vi "MSScript_Calc_GetCmdType.vi"(2 "element":string) -> (1 "Param Items":i32, 4 "SetArray?":bool, 5 "Type":T1)   [LabVIEW 2018, in "MSScript.lvclass"]
uses:
  MSScript.lvclass
  CalcCmdType.ctl
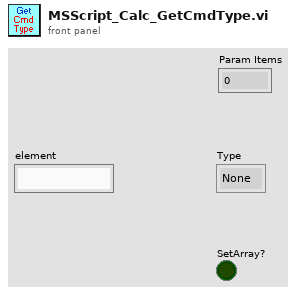
[diagram p1: front panel]
types:
  T1 = typedef "CalcCmdType.ctl" = enum16{"None", "Add", "Sub", "Multiply", "Div", "Pow", "Mod", "Floor", "Ceil", "Round", "Abs", "Sign", "Max", "Min", "mathieu.mz", "mathieu.freq", "mathieu.amp", "mathieu.beta", "ArrayAdd", "ArraySub", "ArrayMultiply", "ArrayDiv", "ArrayPow", "ArrayRoot", "ArrayInit", "ArraySeries", "ArrayLen", "ArraySum"}
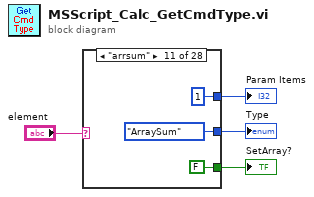
[diagram p0: block diagram]
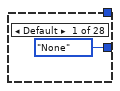
[diagram p2: hidden frame]
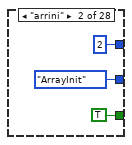
[diagram p3: hidden frame]
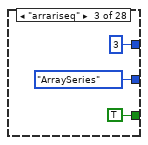
[diagram p4: hidden frame]
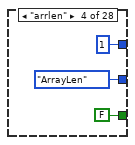
[diagram p5: hidden frame]
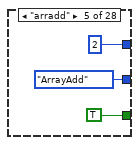
[diagram p6: hidden frame]
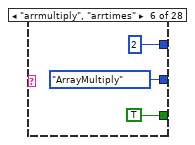
[diagram p7: hidden frame]
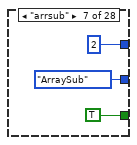
[diagram p8: hidden frame]
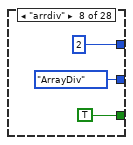
[diagram p9: hidden frame]
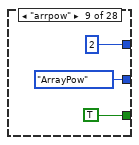
[diagram p10: hidden frame]
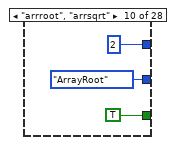
[diagram p11: hidden frame]
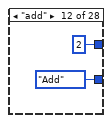
[diagram p12: hidden frame]
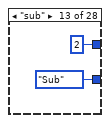
[diagram p13: hidden frame]
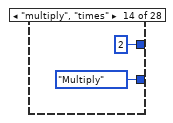
[diagram p14: hidden frame]
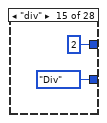
[diagram p15: hidden frame]
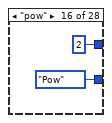
[diagram p16: hidden frame]
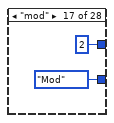
[diagram p17: hidden frame]
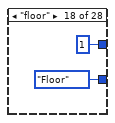
[diagram p18: hidden frame]
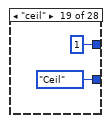
[diagram p19: hidden frame]
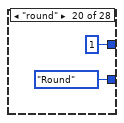
[diagram p20: hidden frame]
diagram:
  n1 = case shown="\"arrsum\"" "element" {
    tunnel: [CalcCmdType."None" ("Type") CalcCmdType."ArrayInit" ("Type") CalcCmdType."ArraySeries" ("Type") CalcCmdType."ArrayLen" ("Type") CalcCmdType."ArrayAdd" ("Type") CalcCmdType."ArrayMultiply" ("Type") CalcCmdType."ArraySub" ("Type") CalcCmdType."ArrayDiv" ("Type") CalcCmdType."ArrayPow" ("Type") CalcCmdType."ArrayRoot" ("Type") CalcCmdType."ArraySum" ("Type") CalcCmdType."Add" ("Type") CalcCmdType."Sub" ("Type") CalcCmdType."Multiply" ("Type") CalcCmdType."Div" ("Type") CalcCmdType."Pow" ("Type") CalcCmdType."Mod" ("Type") CalcCmdType."Floor" ("Type") CalcCmdType."Ceil" ("Type") CalcCmdType."Round" ("Type") CalcCmdType."Abs" ("Type") CalcCmdType."Sign" ("Type") CalcCmdType."Max" ("Type") CalcCmdType."Min" ("Type") CalcCmdType."mathieu.mz" ("Type") CalcCmdType."mathieu.freq" ("Type") CalcCmdType."mathieu.amp" ("Type") CalcCmdType."mathieu.beta" ("Type")] -> w3
    tunnel: [_ TRUE TRUE FALSE TRUE TRUE TRUE TRUE TRUE TRUE FALSE _ _ _ _ _ _ _ _ _ _ _ _ _ _ _ _ _] -> w2
    tunnel: [_ 2 3 1 2 2 2 2 2 2 1 2 2 2 2 2 2 1 1 1 1 1 2 2 3 3 3 3] -> w1
    frame Default {
    }
    frame "arrini" {
    }
    frame "arrariseq" {
    }
    frame "arrlen" {
    }
    frame "arradd" {
    }
    frame "arrmultiply", "arrtimes" {
    }
    frame "arrsub" {
    }
    frame "arrdiv" {
    }
    frame "arrpow" {
    }
    frame "arrroot", "arrsqrt" {
    }
    frame "arrsum" {
    }
    frame "add" {
    }
    frame "sub" {
    }
    frame "multiply", "times" {
    }
    frame "div" {
    }
    frame "pow" {
    }
    frame "mod" {
    }
    frame "floor" {
    }
    frame "ceil" {
    }
    frame "round" {
    }
    frame "abs" {
    }
    frame "sign" {
    }
    frame "max" {
    }
    frame "min" {
    }
    frame "mathieu.mz" {
    }
    frame "mathieu.freq" {
    }
    frame "mathieu.amp" {
    }
    frame "mathieu.beta" {
    }
  }
  "Type" <- w3
  "SetArray?" <- w2
  "Param Items" <- w1
